vi "Data_raw-open.vi"(8 "error in":errorcluster, 11 "file (use dialog)":path) -> (0 "error out":errorcluster, 1 "timedelays":dbl[](array[numeric]), 2 "Raw data":i32[][][][](array[numeric]), 3 "waves":dbl[](array[numeric]), 4 "Trabs precalc":dbl[][](array[numeric]))   [LabVIEW 2019]
panel:
  out "Exp data graph":dbl[][](graph)
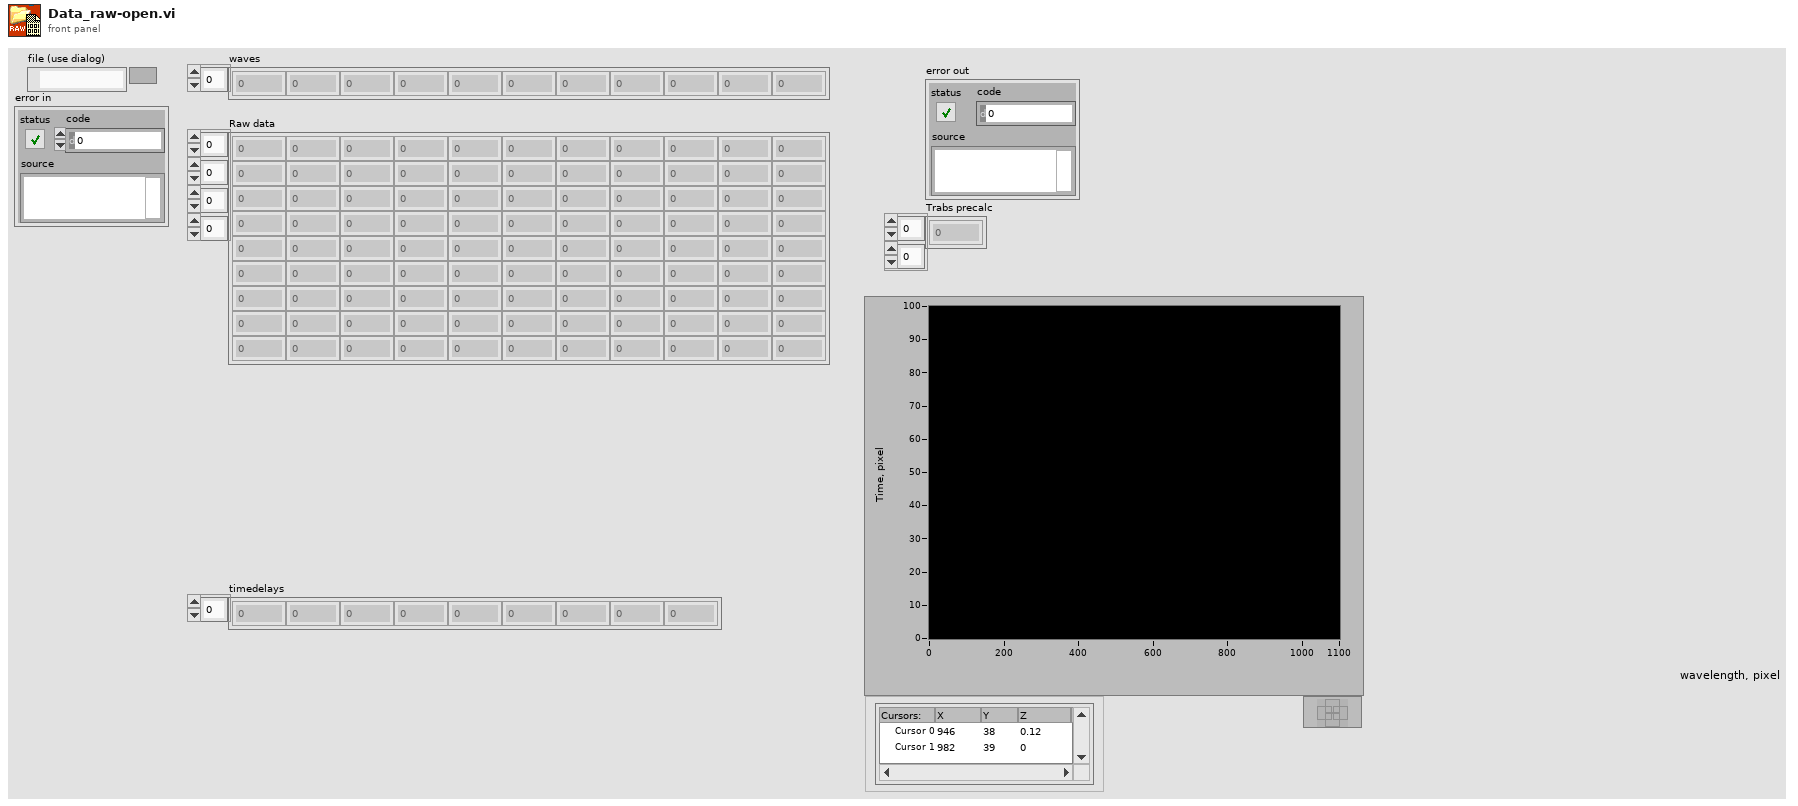
[diagram p1: front panel]
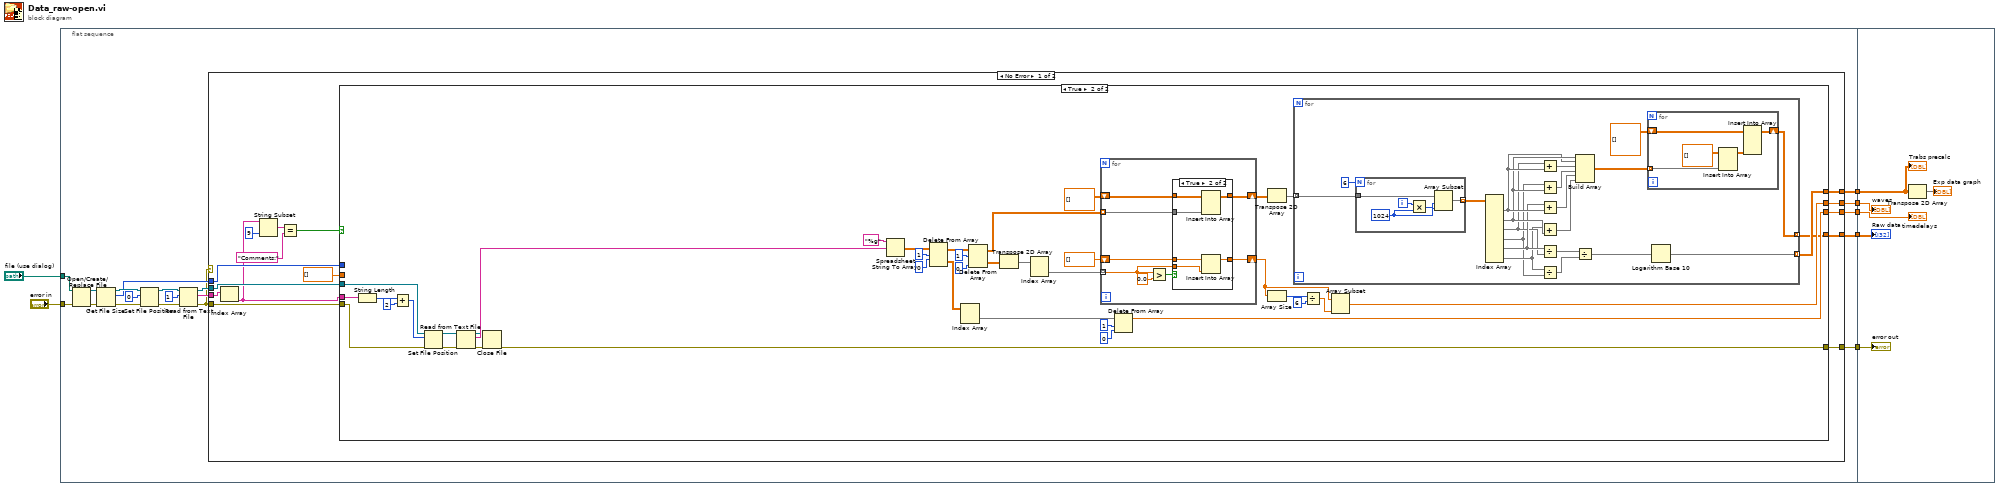
[diagram p0: block diagram]
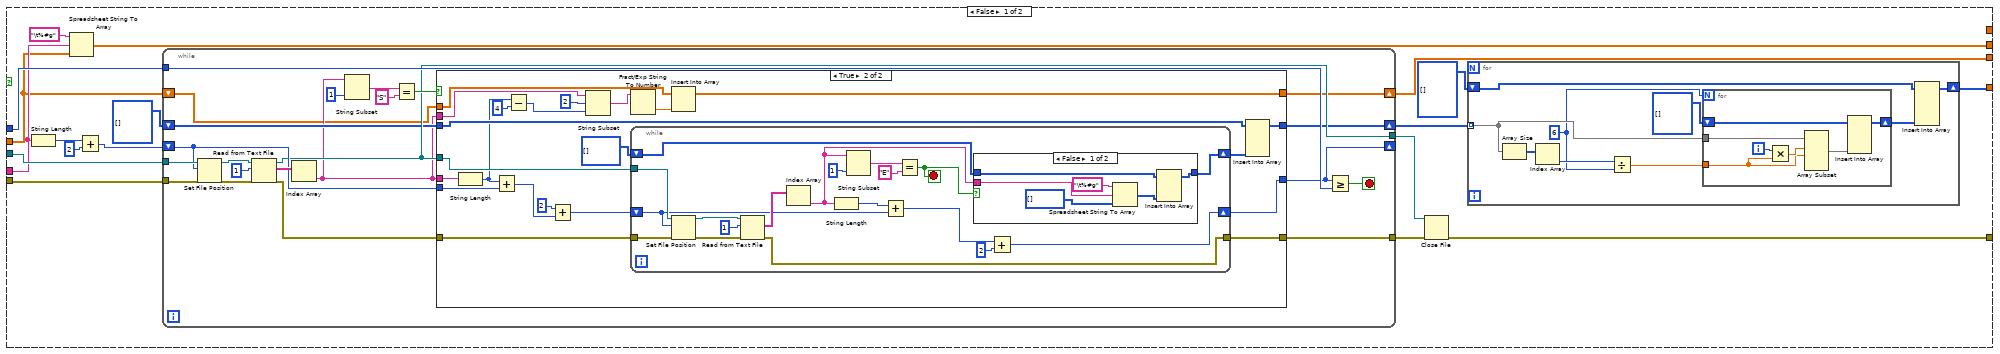
[diagram p2: hidden frame]
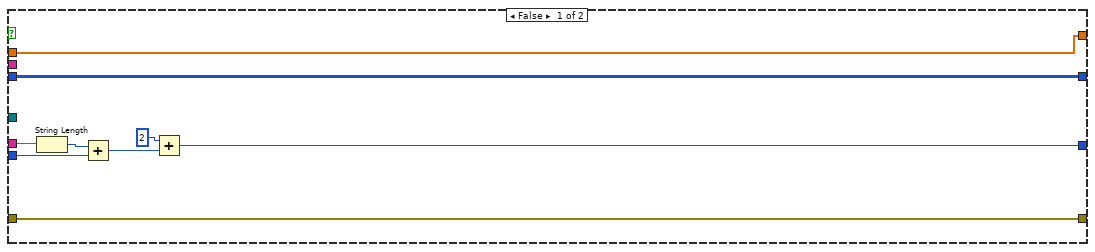
[diagram p3: hidden frame]
diagram:
  n1 = flat-sequence {
    tunnel: "file (use dialog)" -> [w26]
    tunnel: [w14] -> w7
    tunnel: [w13] -> w6
    tunnel: [w12] -> w5
    tunnel: [w11] -> w3
    tunnel: "error in" -> [w10]
    tunnel: [w8] -> w1
    tunnel: w7 -> [w246]
    tunnel: w6 -> [w241]
    tunnel: w5 -> [w245]
    tunnel: w3 -> [w244]
    tunnel: w1 -> [w242]
    frame #0 {
      n2 = Open/Create/Replace File(file path (use dialog)=w26, error in=w10) -> (refnum out=w23:refnum<file>, error out=w24:errorcluster)  [unwired: 4 in, 1 out]
      n3 = Get File Size(file=w23, error in=w24) -> (refnum out=w22:refnum<file>, size (in bytes)=w20:i64, 0:w21:errorcluster)
      n4 = Set File Position(offset (in bytes) (0)=i64 0, refnum=w22, error in=w21) -> (refnum out=w16:refnum<file>, error out=w19:errorcluster)  [unwired: 1 in]
      n5 = Read from Text File(file (use dialog)=w16, count=1, error in=w19) -> (refnum out=w15:refnum<file>, text=w17:string[], error out=w9:errorcluster)  [unwired: 1 in, 1 out]
      n6 = case shown="No Error" w9 {
        selector: w9 -> [_ w240]
        tunnel: w20 -> [w41 _]
        tunnel: w9 -> [w40 _]
        tunnel: w17 -> [w28 _]
        tunnel: w15 -> [w39 _]
        tunnel: [w38 _] -> w14
        tunnel: [w37 _] -> w13
        tunnel: [w36 _] -> w12
        tunnel: [w35 w240] -> w11
        tunnel: [w27 _] -> w8
        frame No Error {
          n7 = Index Array(array=w28) -> (element=w34:string)  [unwired: 1 in]
          n8 = String Subset(string=w34, length (rest)=9 ("length (rest)")) -> (substring=w33:string)  [unwired: 1 in]
          n9 = Equal?(x=w33, y="Comments:") -> (x = y?=w30:bool)
          n10 = case shown="True" w30 {
            tunnel: w41 -> [w59 _]
            tunnel: w40 -> [w58 w190]
            tunnel: w39 -> [w53 w189]
            tunnel: [w47 w162] -> w38
            tunnel: [w42 w181] -> w37
            tunnel: [w46 w155] -> w36
            tunnel: [w45 w157] -> w35
            tunnel: w34 -> [w44 w191]
            tunnel: dbl[] [] ("array type (2D Dbl)") -> [w43 _]
            tunnel: [_ w159] -> w27
            frame False {
              n11 = String Length(string=w44) -> (length=w57:i32)
              n12 = Spreadsheet String To Array(format string="\t%#g", spreadsheet string=w44, array type (2D Dbl)=w43) -> (array=w47:dbl[])  [unwired: 1 in]
              n13 = Add(x=w57, y=2) -> (x+y=w55:i32)
              n14 = while {
                tunnel: w53 -> [w87]
                tunnel: w58 -> [w86]
                shift-right: [w85] -> _
                shift-left: w55 -> [w84]
                tunnel: w59 -> [w95]
                tunnel: [w83] -> w52
                shift-right: [w80] -> w50
                shift-left: i32[][][] [] ("RAW dara") -> [w81]
                shift-right: [w77] -> w42
                shift-left: w43 -> [w78]
                tunnel: [w76] -> w48
                stop <- w94 stop-if-true
                n15 = Set File Position(offset (in bytes) (0)=w84, refnum=w87, error in=w86) -> (refnum out=w88:refnum<file>, error out=w89:errorcluster)  [unwired: 1 in]
                n16 = Read from Text File(file (use dialog)=w88, count=1, error in=w89) -> (refnum out=w83:refnum<file>, text=w97:string[], error out=w82:errorcluster)  [unwired: 1 in, 1 out]
                n17 = Index Array(array=w97) -> (element=w79:string)  [unwired: 1 in]
                n18 = String Subset(string=w79, length (rest)=1 ("length (rest)")) -> (substring=w92:string)  [unwired: 1 in]
                n19 = Equal?(x=w92, y="S") -> (x = y?=w90:bool)
                n20 = case shown="True" w90 {
                  tunnel: w79 -> [w101 w126]
                  tunnel: [w103 w120] -> w85
                  tunnel: w84 -> [w102 w125]
                  tunnel: w83 -> [_ w122]
                  tunnel: w82 -> [w98 w123]
                  tunnel: w81 -> [w100 w119]
                  tunnel: [w100 w118] -> w80
                  tunnel: w79 -> [_ w116]
                  tunnel: [w99 w108] -> w77
                  tunnel: w78 -> [w99 w110]
                  tunnel: [w98 w107] -> w76
                  frame False {
                    n21 = String Length(string=w101) -> (length=w104:i32)
                    n22 = Add(x=w104, y=w102) -> (x+y=w105:i64)
                    n23 = Add(x=i64 2, y=w105) -> (x+y=w103:i64)
                  }
                  frame True {
                    n24 = String Length(string=w126) -> (length=w114:i32)
                    n25 = Add(x=w114, y=w125) -> (x+y=w127:i64)
                    n26 = Subtract(x=w114, y=4) -> (x-y=w112:i32)
                    n27 = Add(x=i64 2, y=w127) -> (x+y=w124:i64)
                    n28 = String Subset(string=w116, offset (0)=2, length (rest)=w112) -> (substring=w111:string)
                    n29 = Fract/Exp String To Number(string=w111) -> (number=w109:dbl)  [unwired: 3 in, 1 out]
                    n30 = while {
                      shift-right: [w135] -> w120
                      shift-left: w124 -> [w133]
                      tunnel: w123 -> [w147]
                      tunnel: w122 -> [w146]
                      shift-right: [w131] -> w117
                      shift-left: i32[][] [] -> [w132]
                      tunnel: [w129] -> w107
                      stop <- w138 stop-if-true
                      n31 = Set File Position(offset (in bytes) (0)=w133, refnum=w146, error in=w147) -> (refnum out=w143:refnum<file>, error out=w144:errorcluster)  [unwired: 1 in]
                      n32 = Read from Text File(file (use dialog)=w143, count=1, error in=w144) -> (text=w142:string[], error out=w129:errorcluster)  [unwired: 1 in, 2 out]
                      n33 = Index Array(array=w142) -> (element=w130:string)  [unwired: 1 in]
                      n34 = String Length(string=w130) -> (length=w137:i32)
                      n35 = String Subset(string=w130, length (rest)=1 ("length (rest)")) -> (substring=w140:string)  [unwired: 1 in]
                      n36 = Add(x=w137, y=w133) -> (x+y=w136:i64)
                      n37 = Equal?(x=w140, y="E") -> (x = y?=w138:bool)
                      n38 = case shown="False" w138 {
                        tunnel: w130 -> [w152 _]
                        tunnel: w132 -> [w149 w154]
                        tunnel: [w148 w154] -> w131
                        frame False {
                          n39 = Spreadsheet String To Array(format string="\t%#g", spreadsheet string=w152, array type (2D Dbl)=i32[] []) -> (array=w150:i32[])  [unwired: 1 in]
                          n40 = Insert Into Array(array=w149, new element=w150) -> (w148:i32[][])  [unwired: 2 in]
                        }
                        frame True {
                        }
                      }
                      n41 = Add(x=w136, y=2) -> (x+y=w135:i64)
                    }
                    n42 = Insert Into Array(array=w110, new element=w109) -> (w108:dbl[])  [unwired: 1 in]
                    n43 = Insert Into Array(array=w119, new element=w117) -> (w118:i32[][][])  [unwired: 3 in]
                  }
                }
                n44 = Greater Or Equal?(x=w85, y=w95) -> (x >= y?=w94:bool)
              }
              n45 = Close File(refnum=w52, error in=w48) -> (error out=w45:errorcluster)  [unwired: 1 out]
              n46 = for {
                tunnel: w50 -> [w64] mode=indexing
                shift-right: [w67] -> w46
                shift-left: i32[][][][] [] ("output array") -> [w68]
                w62 = 6 ("y")
                n47 = Array Size(array=w64) -> (size(s)=w66:i32[])
                n48 = Index Array(array=w66) -> (element=w65:i32)  [unwired: 1 in]
                n49 = Divide(x=w65, y=w62) -> (x/y=w63:dbl)
                n50 = for {
                  N: w62 -> [_]
                  tunnel: w64 -> [w75]
                  tunnel: w63 -> [w72]
                  shift-right: [w69] -> w60
                  shift-left: i32[][][] [] -> [w71]
                  i -> [w74]
                  n51 = Multiply(x=w74, y=w72) -> (x*y=w73:dbl)
                  n52 = Array Subset(array=w75, index (row)=w73, length (row)=w72) -> (w70:i32[][])  [unwired: 2 in]
                  n53 = Insert Into Array(array=w71, new element=w70) -> (w69:i32[][][])  [unwired: 3 in]
                }
                n54 = Insert Into Array(array=w68, new element=w60) -> (w67:i32[][][][])  [unwired: 4 in]
              }
            }
            frame True {
              n55 = String Length(string=w191) -> (length=w193:i32)
              n56 = Add(x=w193, y=2) -> (x+y=w188:i32)
              n57 = Set File Position(offset (in bytes) (0)=w188, refnum=w189, error in=w190) -> (refnum out=w185:refnum<file>, error out=w184:errorcluster)  [unwired: 1 in]
              n58 = Read from Text File(file (use dialog)=w185, error in=w184) -> (refnum out=w156:refnum<file>, text=w186:string, error out=w158:errorcluster)  [unwired: 2 in, 1 out]
              n59 = Close File(refnum=w156, error in=w158) -> (error out=w157:errorcluster)  [unwired: 1 out]
              n60 = Spreadsheet String To Array(format string="%g", spreadsheet string=w186) -> (array=w180:dbl[][])  [unwired: 2 in]
              n61 = Delete From Array(array=w180, length=1, index (row)=0) -> (deleted portion=w174:dbl[][], array with subset deleted=w171:dbl[][])  [unwired: 1 in]
              n62 = Index Array(array=w174) -> (element=w173:dbl[])  [unwired: 2 in]
              n63 = Delete From Array(array=w171, length=1, index (col)=0 ("disabled index (col)")) -> (deleted portion=w169:dbl[][], array with subset deleted=w176:dbl[][])  [unwired: 1 in]
              n64 = Transpose 2D Array(2D array=w169) -> (transposed array=w168:dbl[][])
              n65 = Index Array(array=w168) -> (element=w172:dbl[])  [unwired: 2 in]
              n66 = for {
                tunnel: w176 -> [w228] mode=indexing
                shift-right: [w227] -> w161
                shift-left: dbl[][] [] -> [w229]
                tunnel: w172 -> [w225] mode=indexing
                shift-right: [w224] -> w166
                shift-left: dbl[] [] ("subarray") -> [w226]
                n67 = Greater?(x=w225, y=0.0) -> (0:w230:bool)
                n68 = case shown="True" w230 {
                  tunnel: w229 -> [w233 w239]
                  tunnel: w228 -> [_ w238]
                  tunnel: [w233 w237] -> w227
                  tunnel: w226 -> [w232 w236]
                  tunnel: w225 -> [_ w235]
                  tunnel: [w232 w234] -> w224
                  frame False {
                  }
                  frame True {
                    n69 = Insert Into Array(array=w239, new element=w238) -> (w237:dbl[][])  [unwired: 2 in]
                    n70 = Insert Into Array(array=w236, new element=w235) -> (w234:dbl[])  [unwired: 1 in]
                  }
                }
              }
              n71 = Delete From Array(array=w173, length=1, index=0) -> (array with subset deleted=w181:dbl[])  [unwired: 1 out]
              n72 = Transpose 2D Array(2D array=w161) -> (transposed array=w160:dbl[][])
              n73 = Array Size(array=w166) -> (size(s)=w165:i32)
              n74 = for {
                tunnel: w160 -> [w213] mode=indexing
                tunnel: [w212] -> w159 mode=indexing
                tunnel: [w194] -> w155 mode=indexing
                n75 = for {
                  N: 6 -> [_]
                  tunnel: w213 -> [w223]
                  tunnel: [w219] -> w210 mode=indexing
                  i -> [w222]
                  w221 = 1024 ("y")
                  n76 = Multiply(x=w222, y=w221) -> (x*y=w220:i32)
                  n77 = Array Subset(array=w223, index=w220, length=w221) -> (w219:dbl[])
                }
                n78 = Index Array(array=w210) -> (element #1=w209:dbl[], element #2=w208:dbl[], element #3=w199:dbl[], element #4=w197:dbl[], element #5=w200:dbl[], element #6=w198:dbl[])  [unwired: 12 in]
                n79 = Add(x=w199, y=w209) -> (x+y=w207:dbl[])
                n80 = Add(x=w197, y=w208) -> (x+y=w206:dbl[])
                n81 = Add(x=w200, y=w209) -> (x+y=w205:dbl[])
                n82 = Add(x=w198, y=w208) -> (x+y=w204:dbl[])
                n83 = Divide(x=w200, y=w199) -> (x/y=w202:dbl[])
                n84 = Divide(x=w198, y=w197) -> (x/y=w201:dbl[])
                n85 = Build Array(w209, w208, w207, w206, w205, w204) -> (w195:dbl[][])
                n86 = Divide(x=w202, y=w201) -> (x/y=w203:dbl[])
                n87 = for {
                  shift-right: [w214] -> w194
                  shift-left: dbl[][][] [] -> [w218]
                  tunnel: w195 -> [w216] mode=indexing
                  n88 = Insert Into Array(array=dbl[][] [], new element=w216) -> (w215:dbl[][])  [unwired: 2 in]
                  n89 = Insert Into Array(array=w218, new element=w215) -> (w214:dbl[][][])  [unwired: 3 in]
                }
                n90 = Logarithm Base 10(1:w203) -> (0:w212:dbl[])
              }
              n91 = Divide(x=w165, y=6) -> (x/y=w163:dbl)
              n92 = Array Subset(array=w166, length=w163) -> (w162:dbl[])  [unwired: 1 in]
            }
          }
        }
        frame Error {
        }
      }
    }
    frame #1 {
      n93 = Transpose 2D Array(2D array=w242) -> (transposed array=→"Exp data graph":dbl[][])
      "waves" <- w246
      "Raw data" <- w245
      "timedelays" <- w241
      "error out" <- w244
      "Trabs precalc" <- w242
    }
  }
